vi "test.vi"() -> ()   [LabVIEW 2023, in "HoneywellScanner.lvlib"]
uses:
  HoneywellScanner.lvlib
  ed4c1e00-1c57-4463-aba7-bc3f8cddaf28.vi
  f80544f0-fbb3-49b7-825b-8c9776c06297.vi
panel:
  in  "stop":bool
  in  "y":bool
  out "Scanned value":string
  out "Scan OK":bool
  out "error out":errorcluster
  in  "Scanner Port":string
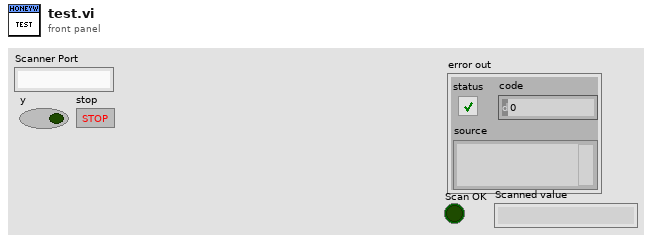
[diagram p1: front panel]
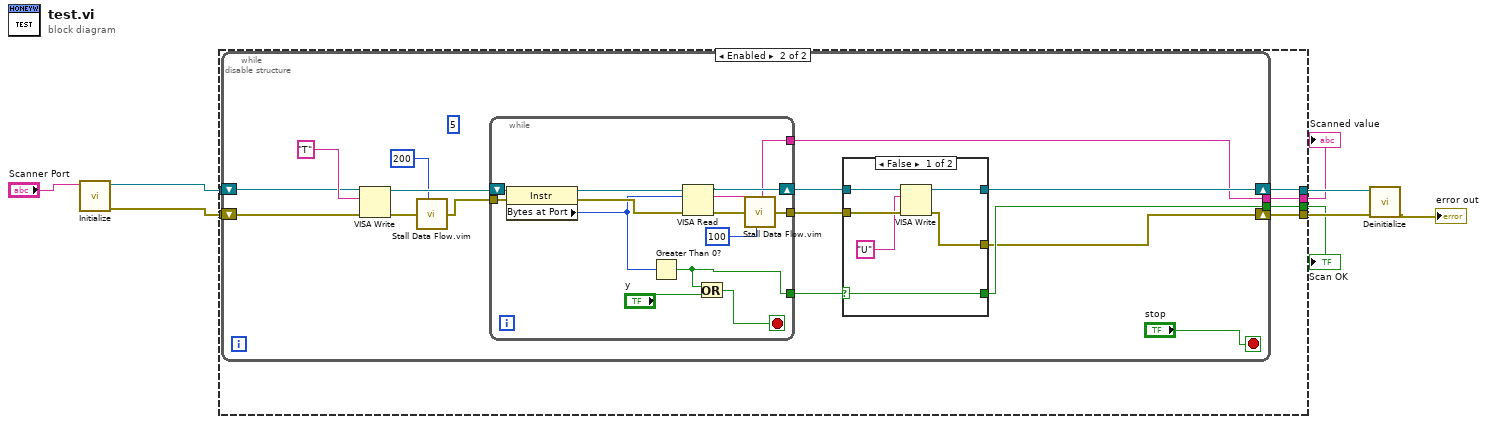
[diagram p0: block diagram]
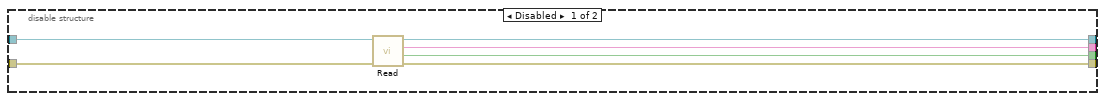
[diagram p2: hidden frame]
diagram:
  n1 = call "Initialize.vi"("Scanner Port"="Scanner Port") -> ("error out"=w6:errorcluster, "Scanner reference"=w1:refnum<visa-resource-name>)  [unwired: 9 in]
  n2 = disable-structure shown="Enabled" {
    disable-tunnel: w1 -> [w14 w15]
    disable-tunnel: [w13 w20] -> w7
    disable-tunnel: w6 -> [w12 w16]
    disable-tunnel: [w11 w17] -> w5
    disable-tunnel: [w10 w18] -> w3
    disable-tunnel: [w9 w19] -> w2
    frame Disabled {
      n3 = call "Read.vi"("error in"=w12, "Scanner reference in"=w14) -> ("error out"=w11:errorcluster, "Scan OK"=w10:bool, "Scanned value"=w9:string, "Scanner reference out"=w13:refnum<visa-resource-name>)  [unwired: 6 in]
    }
    frame Enabled {
      n4 = while {
        tunnel: [w26] -> w19
        tunnel: [w25] -> w18
        shift-right: [w24] -> w17
        shift-left: w16 -> [w23]
        shift-right: [w27] -> w20
        shift-left: w15 -> [w22]
        stop <- "stop" stop-if-true
        (unwired) 5
        n5 = VISA Write(VISA resource name=w22, write buffer="T", error in (no error)=w23) -> (VISA resource name out=w34:refnum<visa-resource-name>, error out=w33:errorcluster)  [unwired: 1 out]
        n6 = call "Stall Data Flow.vim"("value in"=w33, "milliseconds to wait"=u32 200) -> ("value out"=w32:errorcluster)  [unwired: 1 out]
        n7 = while {
          tunnel: w32 -> [w45]
          shift-right: [w44] -> w29
          shift-left: w34 -> [w48]
          tunnel: [w40] -> w28
          tunnel: [w41] -> w26
          tunnel: [w38] -> w30
          stop <- w36 stop-if-true
          n8 = property class="Instr"(reference=w48, error in=w45) -> (reference out=w47:refnum<visa-resource-name>, error out=w46:errorcluster, "Bytes at Port"=w43:u32)
          n9 = Greater Than 0?(x=w43) -> (x > 0?=w38:bool)
          n10 = VISA Read(VISA resource name=w47, byte count=w43, error in (no error)=w46) -> (VISA resource name out=w44:refnum<visa-resource-name>, read buffer=w41:string, error out=w42:errorcluster)  [unwired: 1 out]
          n11 = Or(x=w38, y="y") -> (x .or. y?=w36:bool)
          n12 = call "Stall Data Flow.vim"("value in"=w42, "milliseconds to wait"=u32 100) -> ("value out"=w40:errorcluster)  [unwired: 1 out]
        }
        n13 = case shown="False" w30 {
          selector: w30 -> [w54 w55]
          tunnel: w29 -> [w53 w57]
          tunnel: w28 -> [w51 w56]
          tunnel: [w50 w56] -> w24
          tunnel: [w52 w57] -> w27
          tunnel: [w54 w55] -> w25
          frame False {
            n14 = VISA Write(VISA resource name=w53, write buffer="U", error in (no error)=w51) -> (VISA resource name out=w52:refnum<visa-resource-name>, error out=w50:errorcluster)  [unwired: 1 out]
          }
          frame True {
          }
        }
      }
    }
  }
  "Scan OK" <- w3
  "Scanned value" <- w2
  n15 = call "Deinitialize.vi"("error in (no error)"=w5, "Scanner reference"=w7) -> ("error out"=→"error out":errorcluster)  [unwired: 9 in]
